vi "Mother MRA Saver.vi"(0 "Frequency Saver?":bool, 1 "Dynamic Data":dynamicdata(waveform), 2 "Feature Index":dynamicdata(waveform), 3 "Session Index":dynamicdata(waveform), 4 "Experiment Index":dynamicdata(waveform)) -> ()   [LabVIEW 2023]
uses:
  <vilib>/express/express shared/transition.llb/Dynamic To Waveform Array.vi
  <vilib>/express/express signal manip/GetorSetDDTAttributes/Set DDT Attributes/SetT0.vi
  <vilib>/express/express shared/transition.llb/Waveform Array To Dynamic.vi
  <vilib>/express/express signal manip/GetorSetDDTAttributes/Set DDT Attributes/Set DDT Properties.xnode
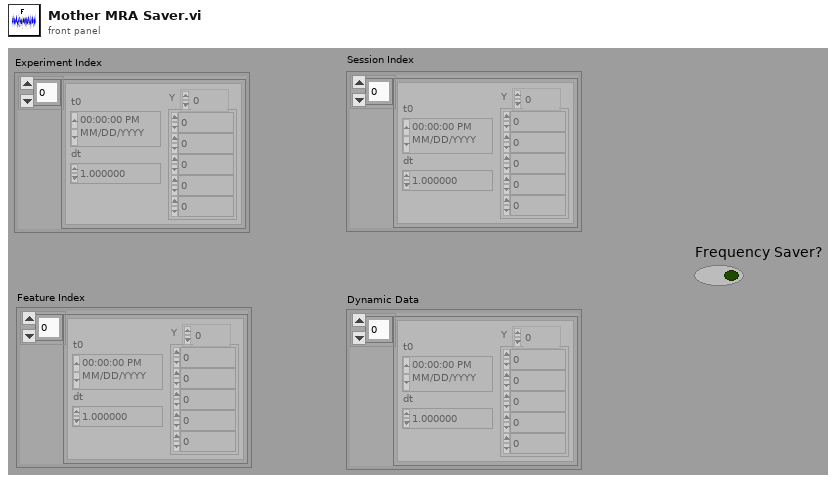
[diagram p1: front panel]
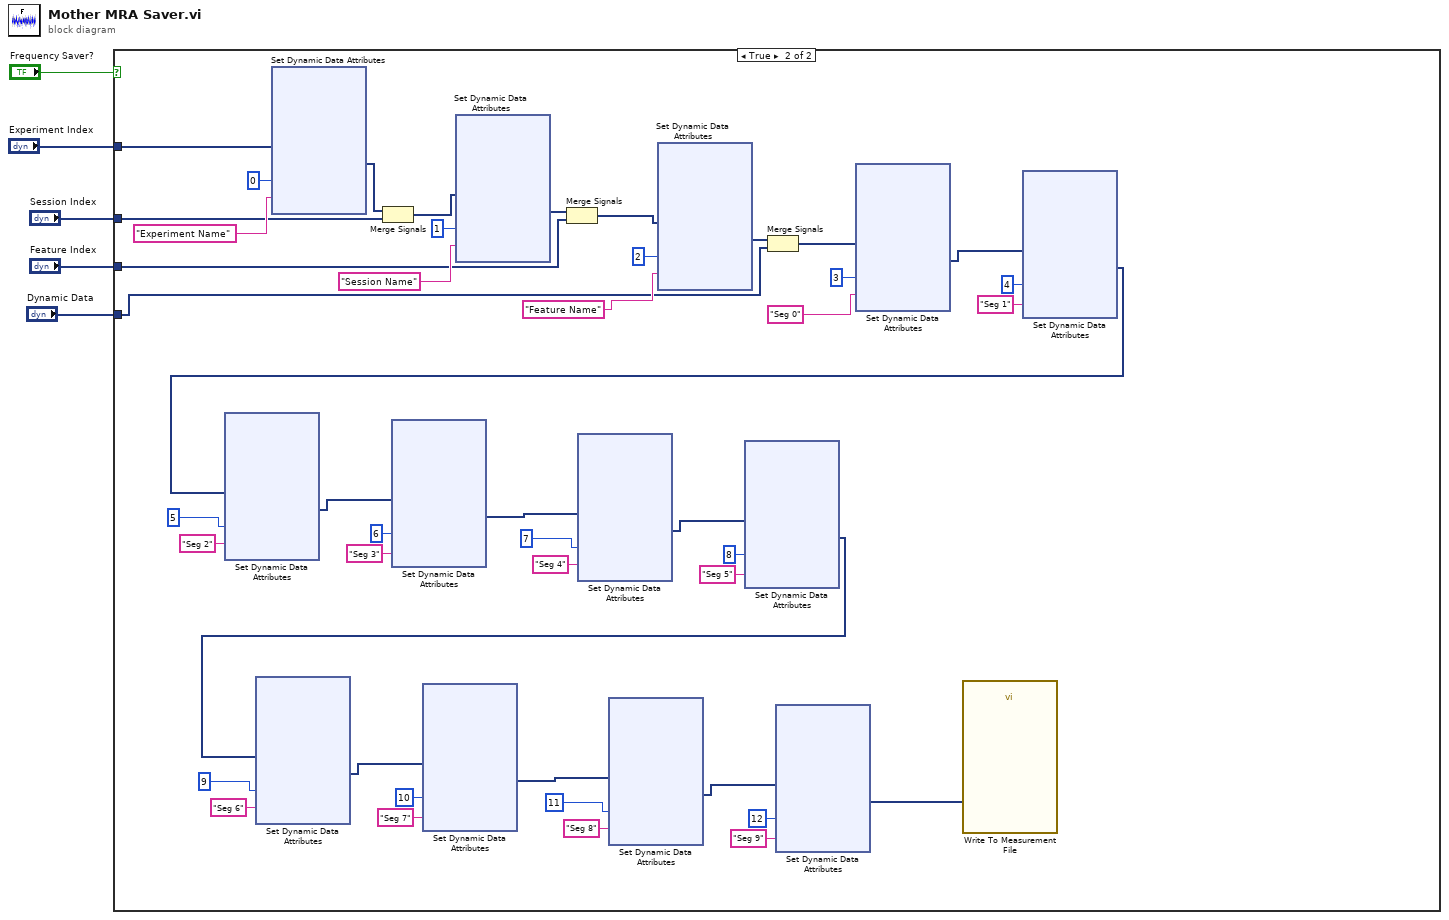
[diagram p0: block diagram]
diagram:
  n1 = case shown="True" "Frequency Saver?" {
    tunnel: "Dynamic Data" -> [_ w34]
    tunnel: "Experiment Index" -> [_ w44]
    tunnel: "Session Index" -> [_ w43]
    tunnel: "Feature Index" -> [_ w35]
    frame False {
    }
    frame True {
      n2 = xnode "Set Dynamic Data Attributes"("Signals In"=w44, "Signal Index"=0, "Signal Name"="Experiment Name") -> ("Signals Out"=w42:dynamicdata)  [unwired: 1 in, 1 out]
      n3 = Merge Signals(w42, w43) -> (w41:dynamicdata)
      n4 = xnode "Set Dynamic Data Attributes"("Signals In"=w41, "Signal Index"=1, "Signal Name"="Session Name") -> ("Signals Out"=w36:dynamicdata)  [unwired: 1 in, 1 out]
      n5 = Merge Signals(w36, w35) -> (w37:dynamicdata)
      n6 = xnode "Set Dynamic Data Attributes"("Signals In"=w37, "Signal Index"=2, "Signal Name"="Feature Name") -> ("Signals Out"=w40:dynamicdata)  [unwired: 1 in, 1 out]
      n7 = Merge Signals(w40, w34) -> (w45:dynamicdata)
      n8 = xnode "Set Dynamic Data Attributes"("Signals In"=w45, "Signal Index"=3, "Signal Name"="Seg 0") -> ("Signals Out"=w33:dynamicdata)  [unwired: 1 in, 1 out]
      n9 = xnode "Set Dynamic Data Attributes"("Signals In"=w33, "Signal Index"=4, "Signal Name"="Seg 1") -> ("Signals Out"=w26:dynamicdata)  [unwired: 1 in, 1 out]
      n10 = xnode "Set Dynamic Data Attributes"("Signals In"=w26, "Signal Index"=5, "Signal Name"="Seg 2") -> ("Signals Out"=w28:dynamicdata)  [unwired: 1 in, 1 out]
      n11 = xnode "Set Dynamic Data Attributes"("Signals In"=w28, "Signal Index"=6, "Signal Name"="Seg 3") -> ("Signals Out"=w19:dynamicdata)  [unwired: 1 in, 1 out]
      n12 = xnode "Set Dynamic Data Attributes"("Signals In"=w19, "Signal Index"=7, "Signal Name"="Seg 4") -> ("Signals Out"=w22:dynamicdata)  [unwired: 1 in, 1 out]
      n13 = xnode "Set Dynamic Data Attributes"("Signals In"=w22, "Signal Index"=8, "Signal Name"="Seg 5") -> ("Signals Out"=w7:dynamicdata)  [unwired: 1 in, 1 out]
      n14 = xnode "Set Dynamic Data Attributes"("Signals In"=w7, "Signal Index"=9, "Signal Name"="Seg 6") -> ("Signals Out"=w10:dynamicdata)  [unwired: 1 in, 1 out]
      n15 = xnode "Set Dynamic Data Attributes"("Signals In"=w10, "Signal Index"=10, "Signal Name"="Seg 7") -> ("Signals Out"=w18:dynamicdata)  [unwired: 1 in, 1 out]
      n16 = xnode "Set Dynamic Data Attributes"("Signals In"=w18, "Signal Index"=11, "Signal Name"="Seg 8") -> ("Signals Out"=w15:dynamicdata)  [unwired: 1 in, 1 out]
      n17 = xnode "Set Dynamic Data Attributes"("Signals In"=w15, "Signal Index"=12, "Signal Name"="Seg 9") -> ("Signals Out"=w6:dynamicdata)  [unwired: 1 in, 1 out]
      n18 = call "Write To Measurement File"("Signals"=w6) -> ()  [unwired: 16 in, 3 out]
    }
  }
